vi "PH_SSAC.evt call set Background Read.vi"(0 "i ref in":refnum<vi>, 1 "Instance":string, 2 "Background Read":bool, 5 "error in (no error)":errorcluster) -> (14 "i ref out":refnum<vi>, 19 "error out":errorcluster)   [LabVIEW 2014, in "PH_SSAC.lvlib"]
doc: "This VI calls an event case by a simple call."
uses:
  PH_SSAC.lvlib
  CSCore/CSSystem/CoreLib/CoreLib.short 2 byte array.vi
  CSCore/CSSystem/CoreLib/CoreLib.lvlib
  CSCore/BaseProcess/BaseProcess.lvlib
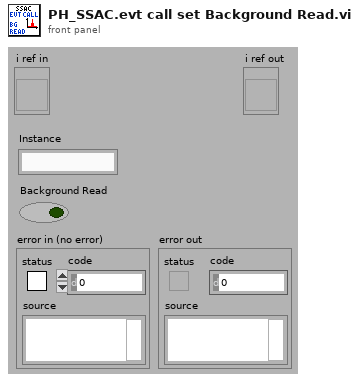
[diagram p1: front panel]
types:
  T1 = typedef "CoreDefs.rawDataType.ctl" = i8[]
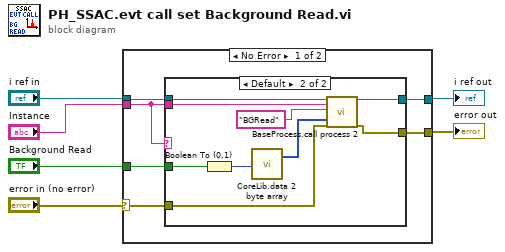
[diagram p0: block diagram]
diagram:
  n1 = case shown="No Error" "error in (no error)" {
    selector: "error in (no error)" -> [w9 w24]
    tunnel: [w12 w25] -> w2
    tunnel: [w11 w24] -> w1
    tunnel: "i ref in" -> [w10 w25]
    tunnel: "Instance" -> [w8 _]
    tunnel: "Background Read" -> [w7 _]
    frame No Error {
      n2 = case shown="Default" w8 {
        tunnel: [w14 w22] -> w12
        tunnel: [w13 w21] -> w11
        tunnel: w10 -> [w14 w20]
        tunnel: w8 -> [_ w19]
        tunnel: w9 -> [w13 w17]
        tunnel: w7 -> [_ w15]
        frame "N/A" {
        }
        frame Default {
          n3 = Boolean To (0,1)(Boolean=w15) -> (0, 1=w16:i16)
          n4 = call-poly "CoreLib.data 2 byte array.vi"("i16"=w16) -> ("byteArray out"=w18:T1)  [unwired: 18 in]
          n5 = call "BaseProcess.call process 2.vi"("i ref in"=w20, "Object"=w19, "Selector"="BGRead", "Data"=w18, "error in (no error)"=w17) -> ("i ref out"=w22:refnum<vi>, "error out"=w21:errorcluster)  [unwired: 13 in]
        }
      }
    }
    frame Error {
    }
  }
  "i ref out" <- w2
  "error out" <- w1
